vi "close_handle.vi"(9 "handle":u64, 11 "path in":path=path "hl2ss_ulm.dll") -> (3 "path out":path)   [LabVIEW 2023]
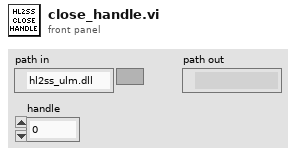
[diagram p1: front panel]
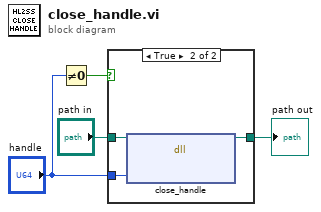
[diagram p0: block diagram]
diagram:
  n1 = Not Equal To 0?(x="handle") -> (x != 0?=w4:bool)
  n2 = case shown="True" w4 {
    tunnel: "path in" -> [w5 w8]
    tunnel: [w5 w7] -> w2
    tunnel: "handle" -> [_ w6]
    frame False {
    }
    frame True {
      n3 = dll-call lib="C:/Users/jcds/Documents/GitHub/hl2ss/extensions/client_labview/hl2ss_ulm.dll" fn="close_handle"(path in=w8, "handle"=w6) -> (path out=w7:path)  [unwired: 4 in, 1 out]
    }
  }
  "path out" <- w2
